vi "RPC__method Query.vi"(8 "error in (no error)":errorcluster, 11 "OOP Server in":refnum<class "Template Server.lvclass">) -> (0 "error out":errorcluster, 3 "OOP Server out":refnum<class "Template Server.lvclass">)   [LabVIEW 2019]
uses:
  Template Server.lvclass
  Template Server.lvclass/Template Server.ctl
  RPC Messages/QueryReponse/QueryResponse_Data.ctl
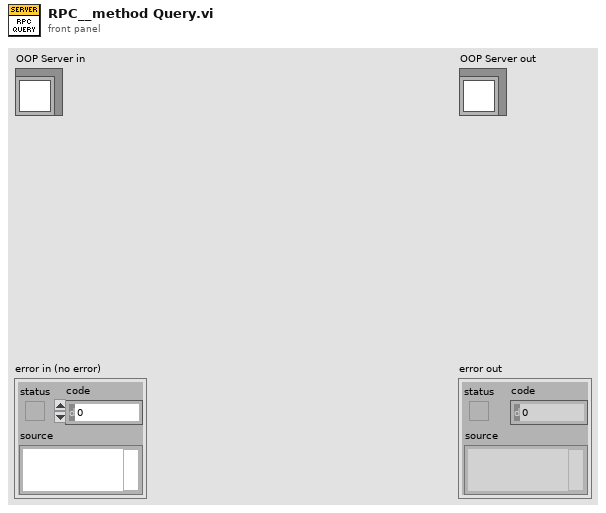
[diagram p1: front panel]
types:
  T1 = typedef "Template Server.lvlib/Template Server.lvclass/QueryResponse_Data.ctl" = cluster{"message":string, "status":i32}
  T2 = typedef "Template Server.lvlib/Template Server.lvclass/Server Internal UEs.ctl" = cluster{"Template Internal UE":refnum<user-event>}
  T3 = typedef "Template Server.lvlib/Template Server.lvclass/Server gRPC UEs.ctl" = cluster{"Template gRPCId UE":T4}
  T4 = typedef "gprc-lvsupport.lvlib/gRPCId Cluster UE.ctl" = refnum<user-event>
  T5 = typedef "gprc-lvsupport.lvlib/grpcId.ctl" = u64
  T6 = typedef "Template Server.lvlib/Template Server.lvclass/QueryRequest_Data.ctl" = cluster{"query":string}
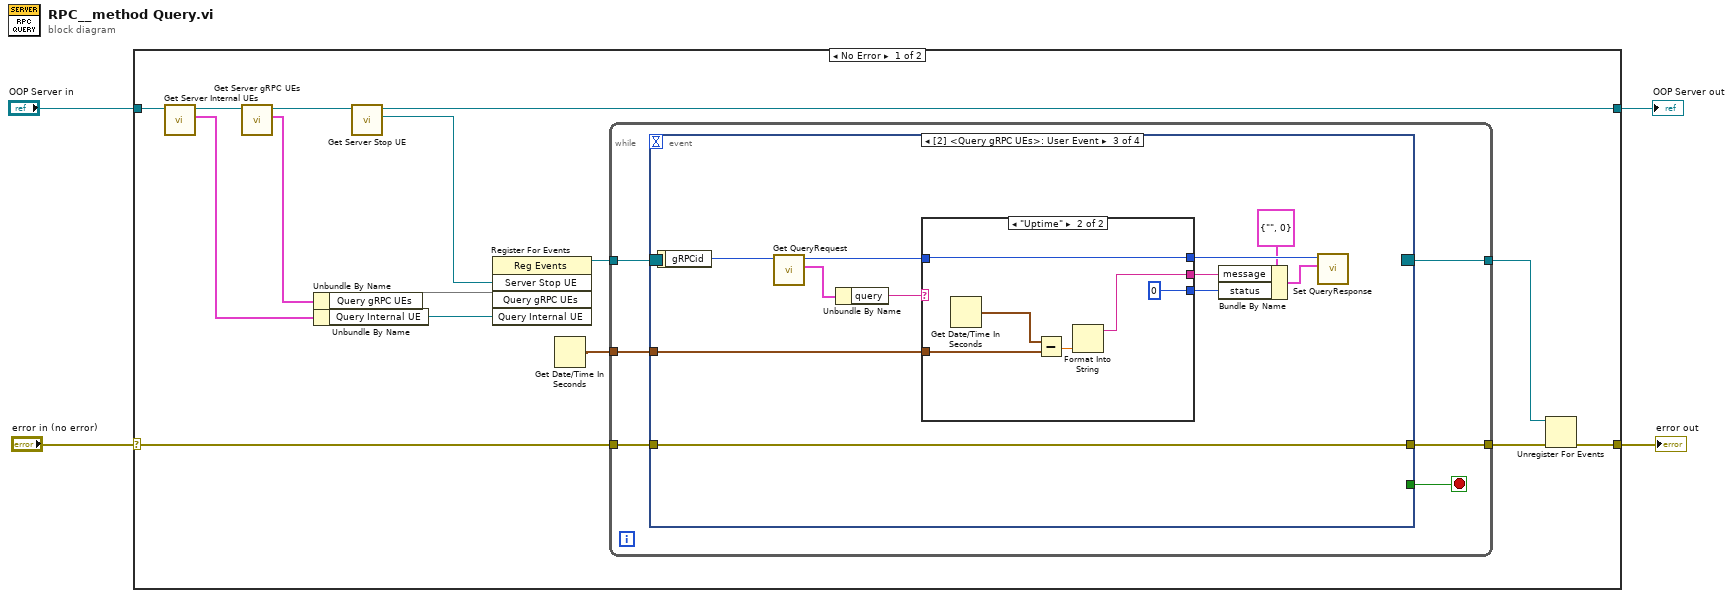
[diagram p0: block diagram]
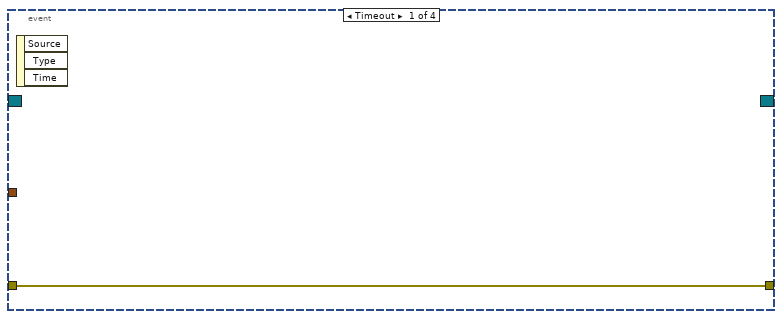
[diagram p2: hidden frame]
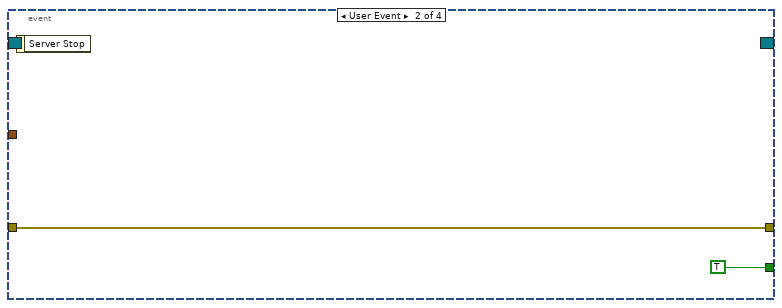
[diagram p3: hidden frame]
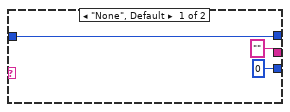
[diagram p4: hidden frame]
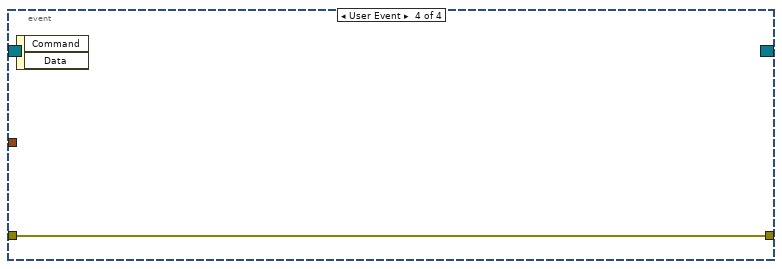
[diagram p5: hidden frame]
diagram:
  n1 = case shown="No Error" "error in (no error)" {
    selector: "error in (no error)" -> [w9 w51]
    tunnel: [w5 w51] -> w3
    tunnel: [w17 w50] -> w1
    tunnel: "OOP Server in" -> [w13 w50]
    frame No Error {
      n2 = call "Get Server Internal UEs.vi"("OOP Server in"=w13) -> ("Server Internal UEs"=w11:T2, "OOP Server out"=w12:refnum<class "Template Server.lvclass">)  [unwired: 9 in]
      n3 = call "Get Server gRPC UEs.vi"("OOP Server in"=w12) -> ("Server gRPC UEs"=w15:T3, "OOP Server out"=w19:refnum<class "Template Server.lvclass">)  [unwired: 9 in]
      n4 = Unbundle By Name(w15) -> ("Query gRPC UEs"=w14)
      n5 = Unbundle By Name(w11) -> ("Query Internal UE"=w10:refnum<user-event>)
      n6 = call "Get Server Stop UE.vi"("OOP Server in"=w19) -> ("Server Stop UE"=w18:refnum<user-event>, "OOP Server out"=w17:refnum<class "Template Server.lvclass">)  [unwired: 9 in]
      n7 = register-events(w18, w14, w10) -> (reference out=w16:refnum<event-registration>)  [unwired: 2 in, 1 out]
      n8 = Get Date/Time In Seconds() -> (seconds since 1Jan1904=w8:timestamp)
      n9 = while {
        tunnel: w16 -> [w25]
        tunnel: w9 -> [w23]
        tunnel: [w22] -> w7
        tunnel: w8 -> [w21]
        tunnel: [w20] -> w6
        stop <- w24 stop-if-true
        n10 = event shown="[2] <Query gRPC UEs>: User Event" {
          selector: w25 -> [_ _ _ _]
          dyn-events: [_ _ _ _] -> w20
          timeout: _ -> [_ _ _ _]
          tunnel: [_ TRUE _ _] -> w24
          tunnel: w23 -> [w26 w27 w39 w49]
          tunnel: [w26 w27 w39 w49] -> w22
          tunnel: w21 -> [_ _ w29 _]
          event Timeout {
            n11 = event-data() -> ()  [unwired: 1 in, 3 out]
          }
          event User Event {
            n12 = event-data() -> ()  [unwired: 1 in, 1 out]
          }
          event User Event {
            n13 = event-data() -> ("gRPCid"=w30:T5)  [unwired: 1 in]
            n14 = call "Get QueryRequest.vi"("gRPCid"=w30) -> ("Request Data"=w38:T6, "gRPCid out"=w36:T5)  [unwired: 8 in, 1 out]
            n15 = Unbundle By Name(w38) -> ("query"=w37:string)
            n16 = case shown="\"Uptime\"" w37 {
              tunnel: w36 -> [w42 w45]
              tunnel: w29 -> [_ w46]
              tunnel: [w42 w45] -> w35
              tunnel: ["" w44] -> w32
              tunnel: [0 ("status") 0 ("status")] -> w31
              frame "None", Default {
              }
              frame "Uptime" {
                n17 = Get Date/Time In Seconds() -> (seconds since 1Jan1904=w48:timestamp)
                n18 = Subtract(x=w48, y=w46) -> (x-y=w47:dbl)
                n19 = Format Into String(w47) -> (resulting string=w44:string)  [unwired: 3 in, 1 out]
              }
            }
            n20 = Bundle By Name(cluster=T1 {"message"="", "status"=0} ("QueryResponse_Data"), "message"=w32, "status"=w31) -> (w33:T1)
            n21 = call "Set QueryResponse.vi"("QueryResponse_Data"=w33, "gRPCid"=w35) -> ()  [unwired: 9 in, 1 out]
          }
          event User Event {
            n22 = event-data() -> ()  [unwired: 1 in, 2 out]
          }
        }
      }
      n23 = Unregister For Events(event registration refnum=w6, error in=w7) -> (error out=w5:errorcluster)
    }
    frame Error {
    }
  }
  "error out" <- w3
  "OOP Server out" <- w1
